vi "Decompose Variant.vi"(8 "error in (no error)":errorcluster, 11 "Variant":variant) -> (0 "error out":errorcluster, 1 "Name":string, 2 "[Name]":string[](array[string]), 3 "[Variant]":variant[](array[variant]))   [LabVIEW 2018, in "Potentiostat Galvanostat.lvclass"]
uses:
  Potentiostat Galvanostat.lvclass
  <vilib>/Utility/Data Type/NI_Data Type.lvlib
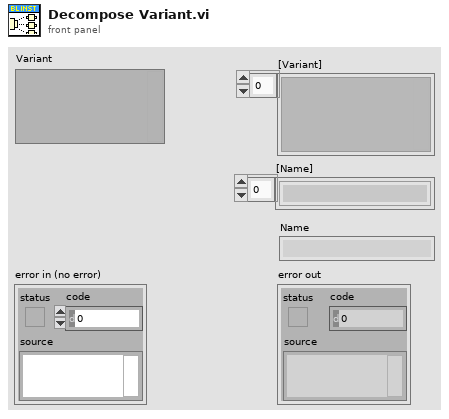
[diagram p1: front panel]
types:
  T1 = typedef "NI_Data Type.lvlib/Data Type.ctl" = enum8{"Invalid Type", "Void", "I8", "I16", "I32", "I64", "U8", "U16", "U32", "U64", "Single Float", "Double Float", "Extended Float", "Single Complex", "Double Complex", "Extended Complex", "Enum U8", "Enum U16", "Enum U32", "Enum U64", "Single Float With Unit", "Double Float With Unit", "Extended Float With Unit", "Single Complex with Unit", "Double Complex with Unit", "Extended Complex with Unit", "Boolean", "String", "Path", "Picture", "Tag", "Array", "Cluster", "Variant", "LV Variant", "Waveform", "Timestamp", "Digital Waveform", "Digital Data", "ExpressData", "Refnum", "External Data", "VI", "Poly VI", "LabVIEW Class Instance", "Fixed Point"}
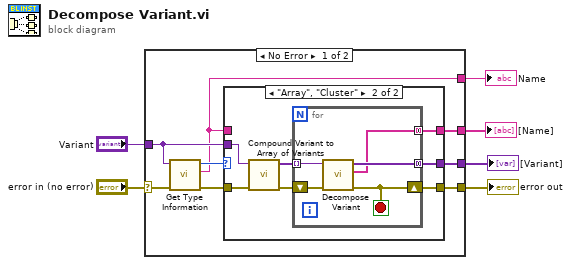
[diagram p0: block diagram]
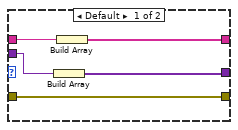
[diagram p2: hidden frame]
diagram:
  n1 = case shown="No Error" "error in (no error)" {
    selector: "error in (no error)" -> [w14 w32]
    tunnel: [w9 w32] -> w5
    tunnel: "Variant" -> [w11 _]
    tunnel: [w10 _] -> w2
    tunnel: [w8 _] -> w3
    tunnel: [w7 _] -> w1
    frame No Error {
      n2 = call <vilib>:"Get Type Information.vi"("error in (no error)"=w14, "Variant"=w11) -> ("error out"=w13:errorcluster, "Name"=w8:string, "Type"=w12:T1)  [unwired: 5 in, 2 out]
      n3 = case shown="\"Array\", \"Cluster\"" w12 {
        tunnel: w13 -> [w19 w26]
        tunnel: w11 -> [w18 w25]
        tunnel: [w19 w22] -> w9
        tunnel: [w17 w21] -> w10
        tunnel: w8 -> [w16 _]
        tunnel: [w15 w20] -> w7
        frame Default {
          n4 = Build Array(w18) -> (w17:variant[])
          n5 = Build Array(w16) -> (w15:string[])
        }
        frame "Array", "Cluster" {
          n6 = call "Compound Variant to Array of Variants.vi"("error in (no error)"=w26, "Array/Cluster Variant"=w25) -> ("error out"=w24:errorcluster, "[Variant]"=w23:variant[])  [unwired: 8 in]
          n7 = for {
            shift-right: [w28] -> w22
            shift-left: w24 -> [w31]
            tunnel: w23 -> [w30] mode=indexing
            tunnel: [w29] -> w21 mode=concatenating
            tunnel: [w27] -> w20 mode=concatenating
            stop <- w28 stop-if-true
            n8 = call "Decompose Variant.vi"("error in (no error)"=w31, "Variant"=w30) -> ("error out"=w28:errorcluster, "[Name]"=w27:string[], "[Variant]"=w29:variant[])  [unwired: 6 in, 1 out]
          }
        }
      }
    }
    frame Error {
    }
  }
  "error out" <- w5
  "Name" <- w3
  "[Variant]" <- w2
  "[Name]" <- w1
